vi "Teleop.vi"(10 "Match Info":T2={"Autonomous Elapsed Seconds"=0.0, "TeleOp Elapsed Seconds"=0.0, "Disabled Elapsed Seconds"=0.0, "Visited Autonomous"=FALSE, "Visited TeleOp"=FALSE, "Visited Disabled"=FALSE, "Autonomous Settings"={"Autonomous Style"=enum."Independent", "VI Refnum"=refnum}}, 11 "Call Context":T3) -> ()   [LabVIEW 2016]
doc: "This VI is called for each TeleOp packet received from the DS where the robot is not disabled. It is often used to read from the joysticks and update I/O or to update setpoints for timed control loops. It should complete and return within 20 milliseconds or it may miss DS packets."
uses:
  <vilib>/Rock Robotics/WPI/DriverStation/WPI_DriverStationDerivedRobotMode.ctl
  <vilib>/Rock Robotics/WPI/DriverStation/WPI_DriverStationMatch Info.ctl
  Robot Global Data.vi
  <vilib>/Rock Robotics/WPI/Utilities/WPI_GetSetVariantRefNum.vi
  <vilib>/Rock Robotics/WPI/Solenoid/Deprecated/WPI_SolenoidSetBool.vi
  <vilib>/Rock Robotics/Network Tables/NT Write Number.vi
  <vilib>/Rock Robotics/Network Tables/NT Write Boolean.vi
  <vilib>/addons/control/pid/pid.llb/PID (DBL).vi
  navX Library v2/navX Library v2.lvlib
  <vilib>/addons/control/pid/NI_PID_pid.lvlib
panel:
  in  "MOE":dbl=25.0 format="%#_13g"
  in  "Center":dbl=180.0 format="%#_13g"
  out "out left":dbl
  out "out right":dbl
  in  "Pid Factor":dbl=8400.0
  in  "Mode":bool=TRUE
  in  "output range":cluster{"output high":dbl, "output low":dbl}={"output high"=1.0, "output low"=-1.0} {"output low" format="%.2f"; "output high" format="%.2f"}
  in  "PID gains":T1={"proportional gain (Kc)"=0.00021, "integral time (Ti, min)"=15.0, "derivative time (Td, min)"=0.0} {"derivative time (Td, min)" format="%.6f"; "integral time (Ti, min)" format="%.6f"; "proportional gain (Kc)" format="%.6f"}
  out "Left":dbl(graph)
  out "Right":dbl(graph)
  out "Encoder Right":dbl(graph)
  out "Encoder Left":dbl(graph)
  in  "Speed":dbl=0.45 format="%#_13g"
  out "Out Left":dbl(graph)
  out "Out Right":dbl(graph)
  out "Shooter":cluster{"Sensor Velocity":dbl, dbl, dbl}(graph)
  in  "ShooterRPM":dbl
  in  "P":dbl=0.5 format="%#_13g"
  in  "I":dbl format="%#_13g"
  in  "D":dbl format="%#_13g"
  in  "F":dbl=0.005212 format="%#_13g"
  in  "I Zone":dbl format="%#_13g"
  in  "Ramp Rate":dbl format="%#_13g"
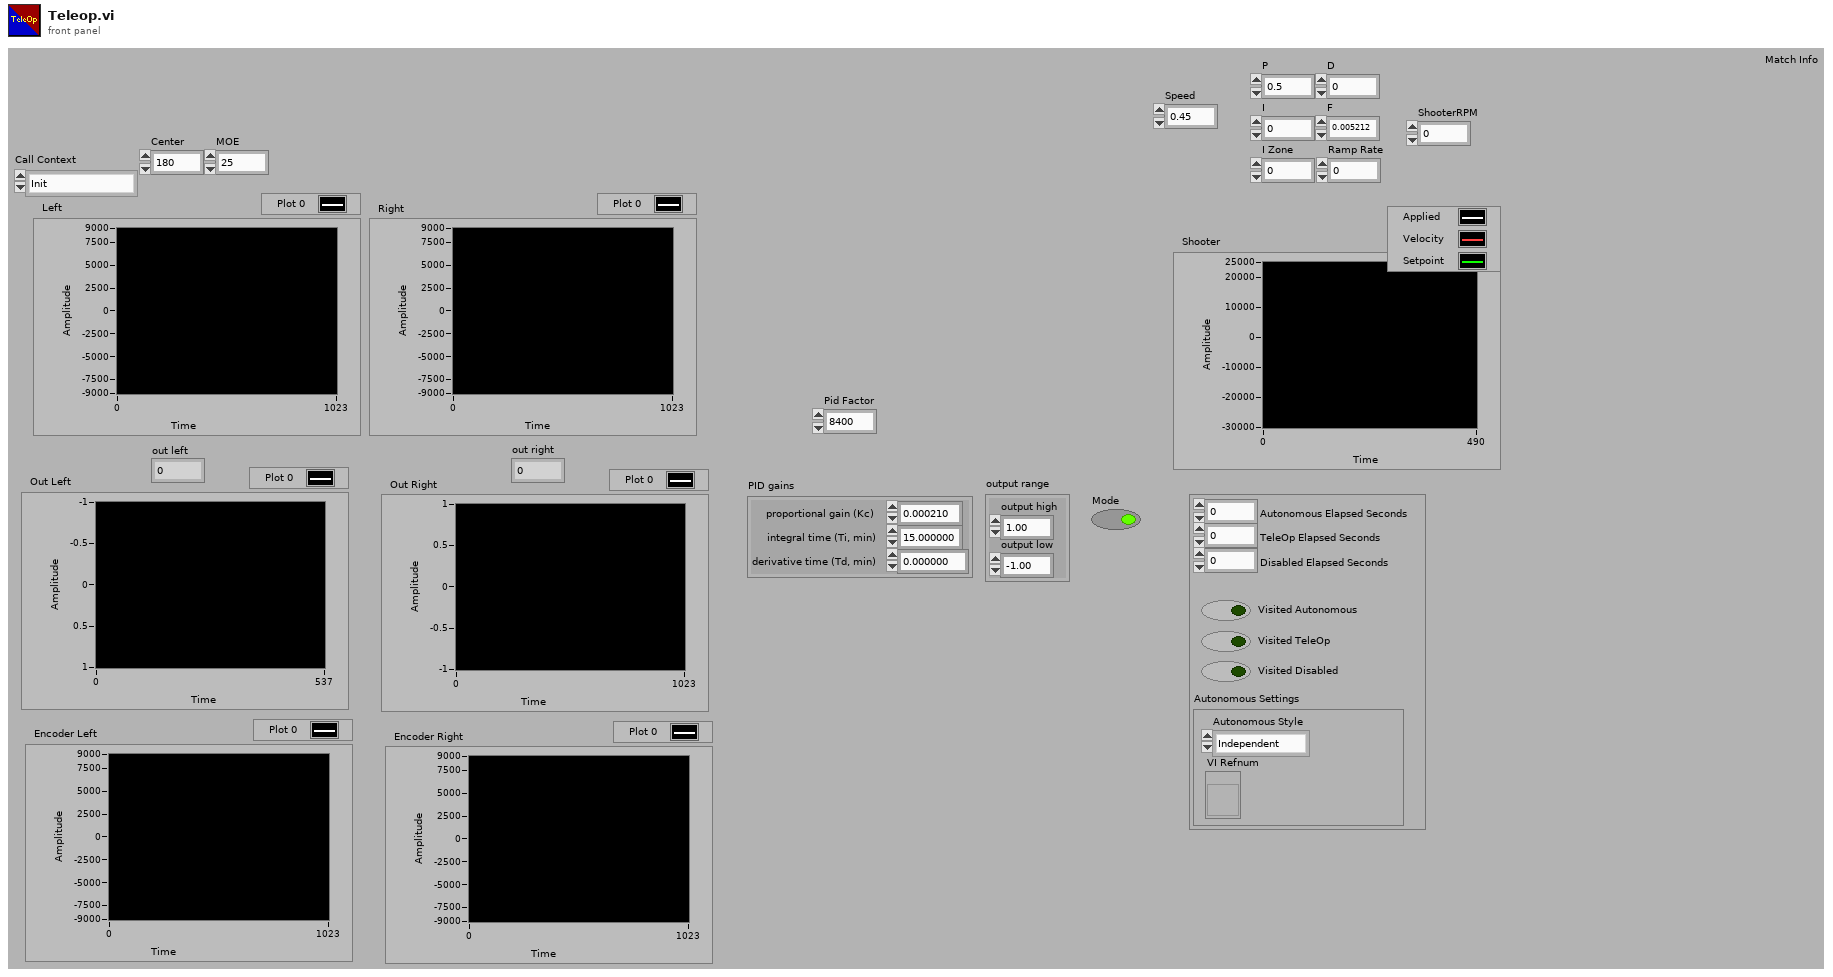
[diagram p1: front panel]
types:
  T1 = cluster{"proportional gain (Kc)":dbl, "integral time (Ti, min)":dbl, "derivative time (Td, min)":dbl}
  T2 = typedef "WPI_DriverStationMatch Info.ctl" = cluster{"Autonomous Elapsed Seconds":dbl, "TeleOp Elapsed Seconds":dbl, "Disabled Elapsed Seconds":dbl, "Visited Autonomous":bool, "Visited TeleOp":bool, "Visited Disabled":bool, "Autonomous Settings":cluster{"Autonomous Style":enum16{"Iterative", "Independent"}, "VI Refnum":refnum<vi>}}
  T3 = typedef "WPI_DriverStationDerivedRobotMode.ctl" = enum16{"Init", "Execute", "Stop"}
  T4 = typedef "WPI_SolenoidDevRef.ctl" = cluster{"DevStatus":errorcluster, "Pneumatics Control Module":u8, "Forward Solenoid Channel":T5, "Reverse Solenoid Channel":T5}
  T5 = typedef "WPI_SolenoidChannel.ctl" = enum8{"Solenoid 0", "Solenoid 1", "Solenoid 2", "Solenoid 3", "Solenoid 4", "Solenoid 5", "Solenoid 6", "Solenoid 7", "Invalid"}
  T6 = typedef "WPI_JoystickDevRef.ctl" = cluster{"Device":T7}
  T7 = typedef "WPI_JoystickDeviceEnum.ctl" = enum16{"USB 0", "USB 1", "USB 2", "USB 3", "USB 4", "USB 5"}
  T8 = cluster{"Buttons[0]":bool, "Buttons[1]":bool, "Buttons[2]":bool, "Buttons[3]":bool, "Buttons[4]":bool, "Buttons[5]":bool, "Buttons[6]":bool, "Buttons[7]":bool, "Buttons[8]":bool}
  T9 = cluster{"Axes[0]":dbl, "Axes[1]":dbl, "Axes[2]":dbl, "Axes[3]":dbl, "Axes[4]":dbl, "Axes[5]":dbl, "Axes[6]":dbl, "Axes[7]":dbl, "Axes[8]":dbl}
  T10 = typedef "navX Library v2.lvlib/Z900_navX_DeviceTypeDef.ctl" = cluster{"Interface":cluster{"Protocol":T11, "Update Rate (4Hz-100Hz)":u8, "navX Open TypeDef":variant}, "Notify Packet":refnum<notifier>, "Loop VI Refnum":refnum<vi>, "Ready to Close Occurrence Refnum":refnum<k4>}
  T11 = typedef "navX Library v2.lvlib/Z900_navX_ProtocolTypeDef.ctl" = enum16{"SERIAL", "I2C", "SPI"}
  T12 = cluster{"Velocity X":dbl, "Velocity Y":dbl, "Velocity Z":dbl, "Displacement X":dbl, "Displacement Y":dbl, "Displacement Z":dbl}
  T13 = cluster{"LinearAcceleration X":dbl, "LinearAcceleration Y":dbl, "LinearAcceleration Z":dbl}
  T14 = cluster{"Yaw":dbl, "Roll":dbl, "Pitch":dbl, "Heading":dbl, "Fused Heading":dbl}
  T15 = typedef "WPI_MotorControlDeviceRef.ctl" = cluster{"DeviceStatus":errorcluster, "Type":T16, "PWM":cluster{"PWM Channel":T17, "DeadBand":T18}, "CAN":cluster{"Device Number":u8, "SetOutput VI Ref":variant, "GetOutput VI Ref":variant, "Enable VI Ref":variant, "Disable VI Ref":variant, "Data":variant}, "Invert":bool}
  T16 = typedef "WPI_MotorControlType.ctl" = enum16{"PWM", "CAN"}
  T17 = typedef "FPGA_DIOPWMChannel.ctl" = enum8{"PWM 0", "PWM 1", "PWM 2", "PWM 3", "PWM 4", "PWM 5", "PWM 6", "PWM 7", "PWM 8", "PWM 9", "PWM MXP 0", "PWM MXP 1", "PWM MXP 2", "PWM MXP 3", "PWM MXP 4", "PWM MXP 5", "PWM MXP 6", "PWM MXP 7", "PWM MXP 8", "PWM MXP 9", "Invalid"}
  T18 = typedef "WPI_PWMDeadband.ctl" = cluster{"Name":string, "maxPositivePwm":i32, "minPositivePwm":i32, "centerPwm":i32, "maxNegativePwm":i32, "minNegativePwm":i32, "angularRange":u16}
  T19 = typedef "WPI_CANTalonSRX_GlobalStatus.ctl" = cluster{"Applied Throttle":dbl, "Module Enabled":bool, "CAN Error":errorcluster, "Closed Loop Error":dbl, "Forward Limit Switch Closed":bool, "Reverse Limit Switch Closed":bool, "Sensor Position":dbl, "Sensor Velocity":dbl, "Current":dbl, "Sticky Fault - Over Temp":bool, "Sticky Fault - Under Voltage":bool, "Sticky Fault - Forward Limit":bool, "Sticky Fault - Reverse Limit":bool, "Sticky Fault - Forward Soft Limit":bool, "Sticky Fault - Reverse Soft Limit":bool, "Brake is Enabled":bool, "Encoder Position":dbl, "Encoder Velocity":dbl, "Encoder Index Count":dbl, "Encoder A Pin State":bool, "Encoder B Pin State":bool, "Encoder Index Pin State":bool, "Analog In":dbl, "Analog In Velocity":dbl, "Temperature (C)":dbl, "Battery Voltage":dbl, "Control 5 Is Supported":bool, "Current Profile Slot Select":dbl, "Pos Div 8":bool, "Vel Div 4":bool, "Pulse Width Position":i32, "Pulse Width Velocity":i32, "Pulse Width Rise To Rise (us)":i32, "Pulse Width Rise To Fall (us)":i32, "Mot Prof Active Is Under Run":bool, "Mot Prof Active Has Under Run":bool, "Mot Prof Active Is Last":bool, "Mot Prof Active Velocity Only":bool, "Mot Prof Active Is Valid":bool, "Mot Prof Buffer Is Full":bool, "Mot Prof Active Profile Slot Select":i32, "Mot Prof NextID":i32, "Mot Prof Count":i32, "Mot Prof Active Velocity":dbl, "Mot Prof Active Position":dbl, "Mot Prof Output Enable":i32}
  T20 = cluster{dbl, "Sensor Velocity":dbl, "ShooterRPM":dbl}
  T21 = typedef "WPI_EncoderDevRef.ctl" = cluster{"DevStatus":errorcluster, "EncoderIndex":T22, "CounterIndex":T23, "DistancePerCount":dbl, "Decoding Type":T24}
  T22 = typedef "FPGA_EncoderIdx.ctl" = enum8{"Enc 0", "Enc 1", "Enc 2", "Enc 3", "Enc 4", "Enc 5", "Enc 6", "Enc 7", "Invalid"}
  T23 = typedef "FPGA_CounterCtrSystemIndex.ctl" = enum8{"Ctr 0", "Ctr 1", "Ctr 2", "Ctr 3", "Ctr 4", "Ctr 5", "Ctr 6", "Ctr 7", "Invalid"}
  T24 = typedef "WPI_EncoderType.ctl" = enum16{"1x", "2x", "4x"}
  T25 = typedef "WPI_RobotDriveDevRef.ctl" = cluster{"DevStatus":errorcluster, "Motors[]":T15[], "Square Inputs":bool, "Max Output":dbl}
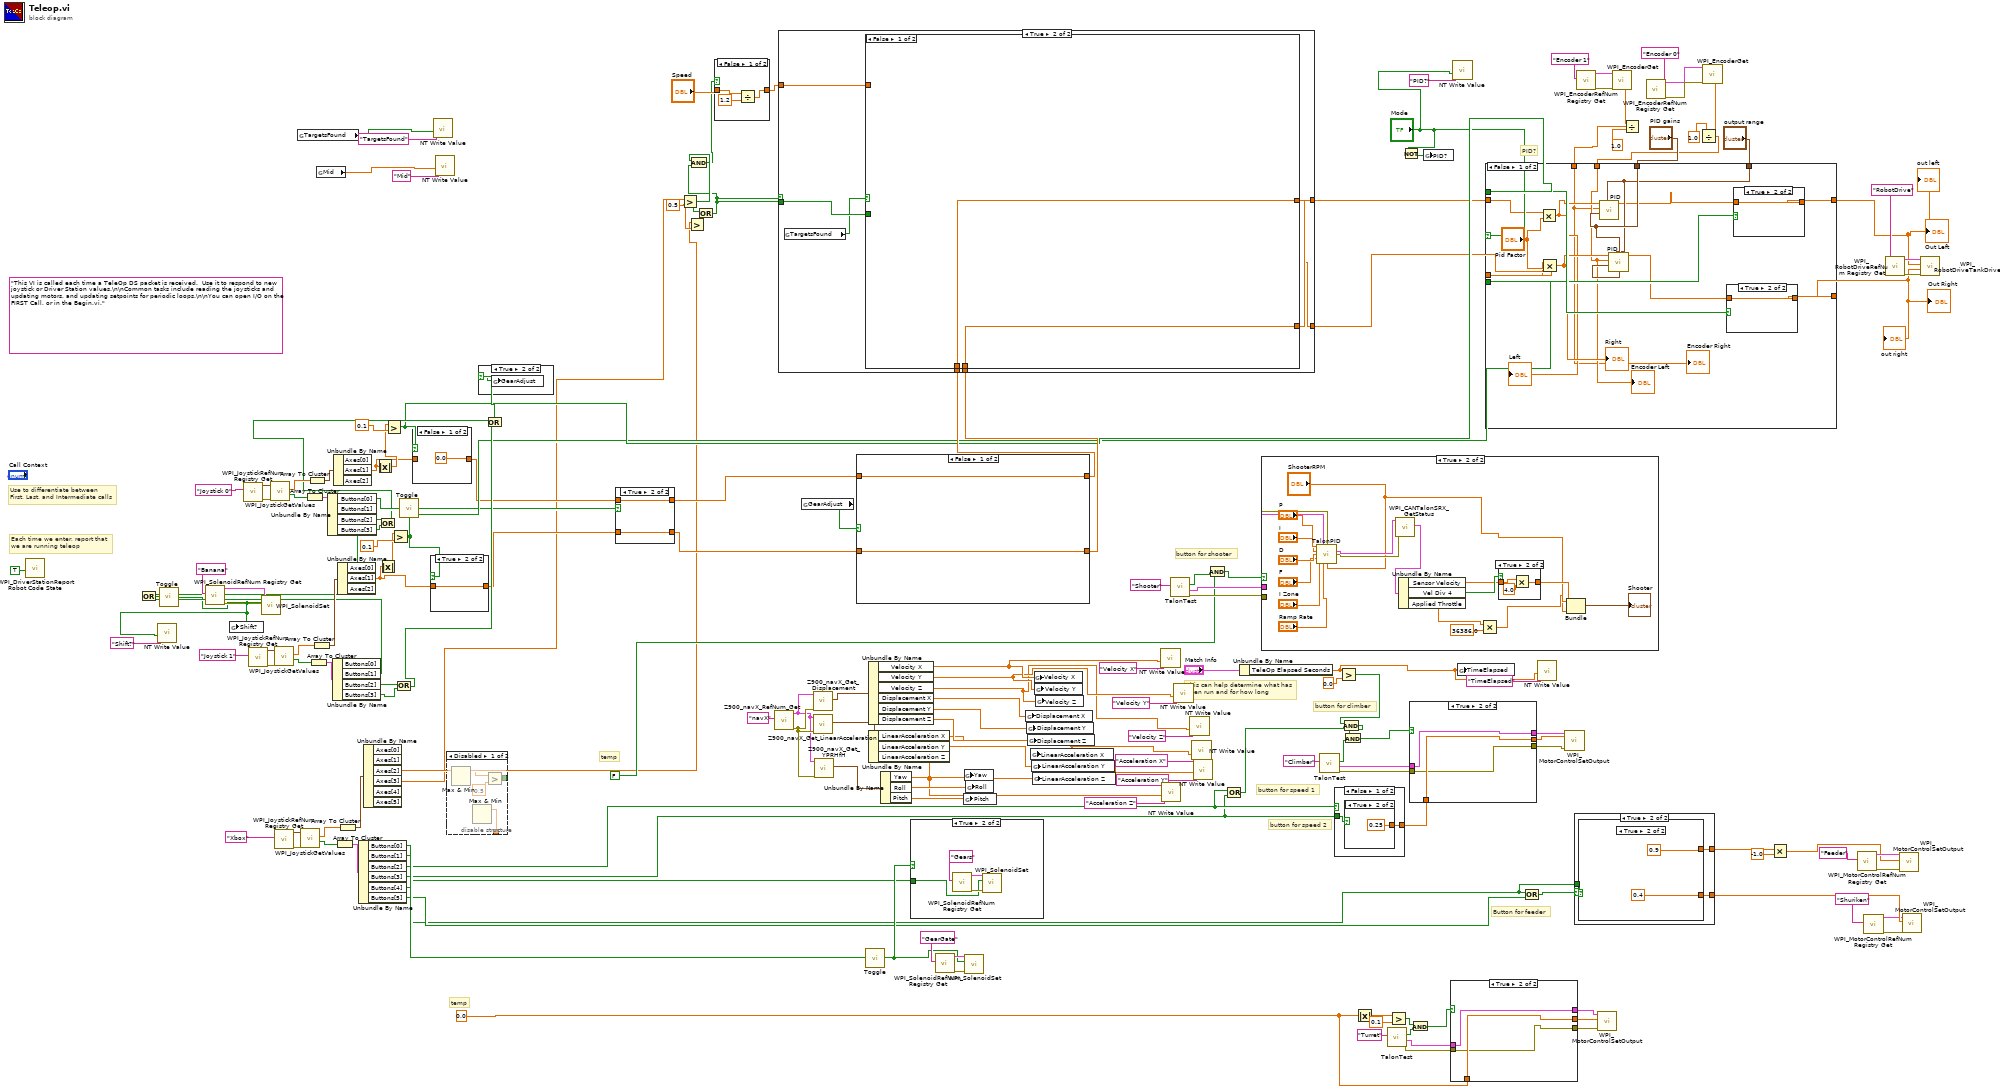
[diagram p0: block diagram]
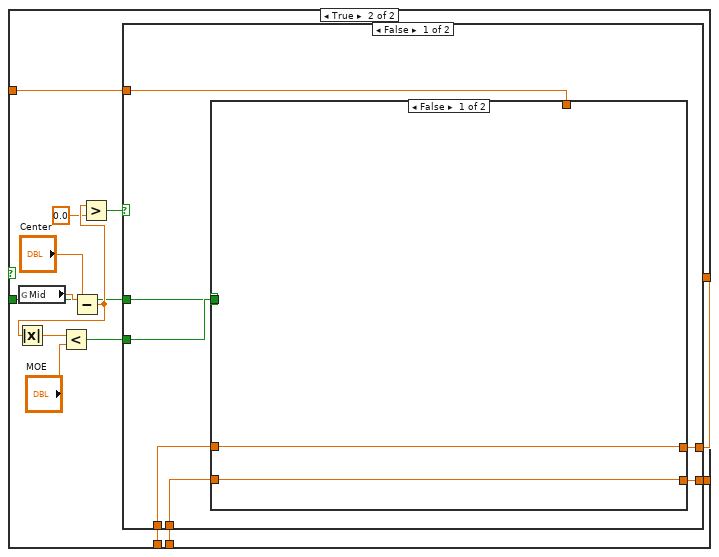
[diagram p4: hidden frame]
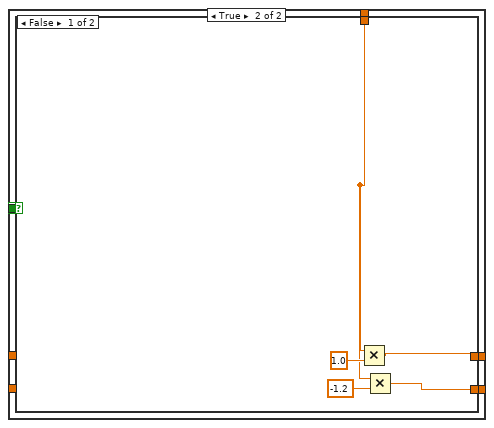
[diagram p5: hidden frame]
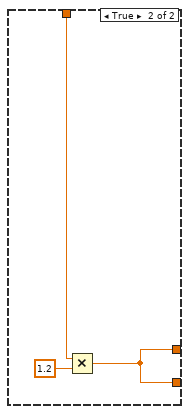
[diagram p6: hidden frame]
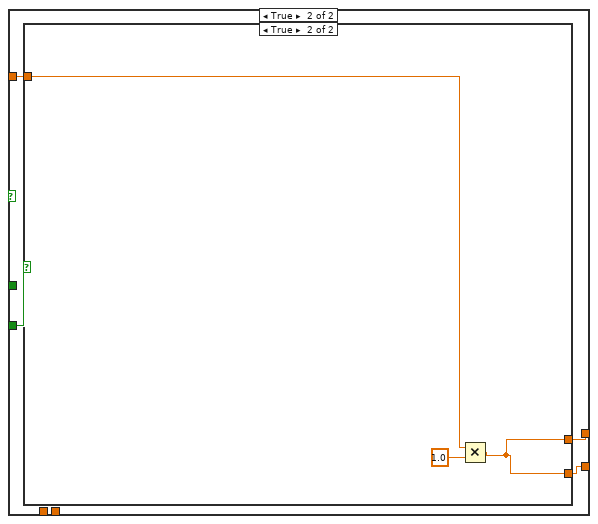
[diagram p7: hidden frame]
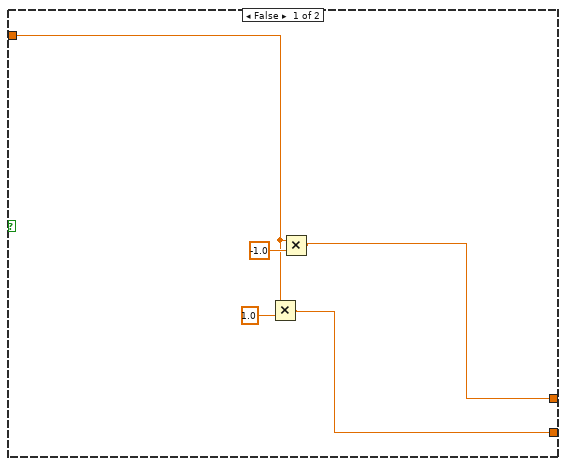
[diagram p8: hidden frame]
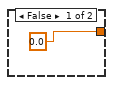
[diagram p9: hidden frame]
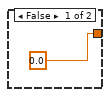
[diagram p10: hidden frame]
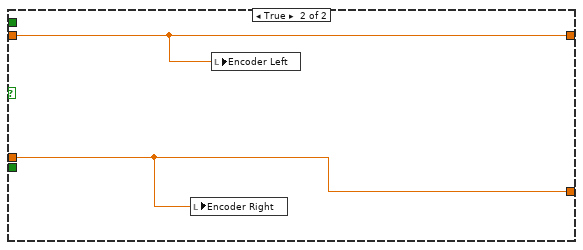
[diagram p11: hidden frame]
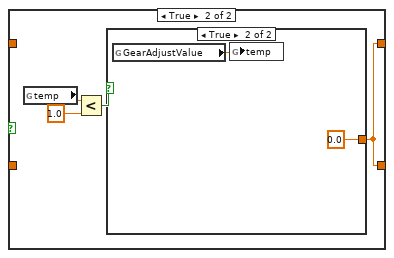
[diagram p14: hidden frame]
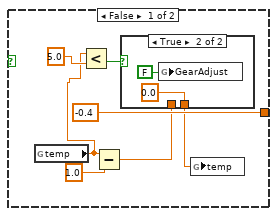
[diagram p15: hidden frame]
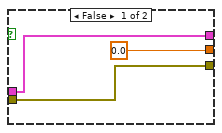
[diagram p17: hidden frame]
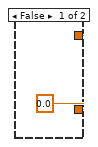
[diagram p19: hidden frame]
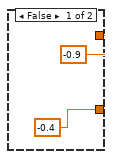
[diagram p20: hidden frame]
diagram:
  w32 = 0.5 ("y")
  w76 = 0.0
  (unwired) "This VI is called each time a TeleOp DS packet is received.  Use it to respond to new joystick or Driver Station values.\n\nCommon tasks include reading the joysticks and updating motors, and updating setpoints for periodic loops.\n\nYou can open I/O on the FIRST Call, or in the Begin.vi."
  # "PID?"
  # "temp"
  # "temp"
  # "Button for feeder"
  # "button for speed 2"
  # "button for speed 1"
  # "button for climber"
  # "button for shooter"
  # "Each time we enter, report that\nwe are running teleop"
  # "Use to differentiate between\nFirst, Last, and Intermediate calls"
  # "This can help determine what has\nbeen run and for how long"
  n1 = call <vilib>:"WPI_DriverStationReport Robot Code State.vi"("TeleOp"=TRUE ("Autonomous")) -> ()  [unwired: 10 in, 1 out]
  n2 = call <vilib>:"WPI_SolenoidRefNum Registry Get.vi"("refnum name"="Banana") -> ("error out"=w40:errorcluster, "SolenoidDevRef"=w39:T4)  [unwired: 9 in]
  n3 = call <vilib>:"WPI_JoystickRefNum Registry Get.vi"("refnum name"="Joystick 0") -> ("error out"=w169:errorcluster, "JoystickDevRef"=w168:T6)  [unwired: 9 in]
  n4 = call <vilib>:"WPI_JoystickRefNum Registry Get.vi"("refnum name"="Joystick 1") -> ("error out"=w161:errorcluster, "JoystickDevRef"=w160:T6)  [unwired: 9 in]
  n5 = call <vilib>:"WPI_JoystickGetValues.vi"("error in (no error)"=w169, "JoystickDevRef"=w168) -> ("Buttons"=w165:bool[], "Axes"=w166:dbl[])  [unwired: 5 in, 3 out]
  n6 = call <vilib>:"WPI_JoystickRefNum Registry Get.vi"("refnum name"="Xbox") -> ("error out"=w123:errorcluster, "JoystickDevRef"=w122:T6)  [unwired: 9 in]
  n7 = call <vilib>:"WPI_JoystickGetValues.vi"("error in (no error)"=w161, "JoystickDevRef"=w160) -> ("Buttons"=w157:bool[], "Axes"=w158:dbl[])  [unwired: 5 in, 3 out]
  n8 = global read "Robot Global Data.vi" "TargetsFound"() -> (w3:bool)
  n9 = call <vilib>:"WPI_JoystickGetValues.vi"("error in (no error)"=w123, "JoystickDevRef"=w122) -> ("Buttons"=w119:bool[], "Axes"=w120:dbl[])  [unwired: 5 in, 3 out]
  n10 = Array To Cluster(array=w165) -> (cluster=w163:T8)
  n11 = Array To Cluster(array=w166) -> (cluster=w164:T9)
  n12 = Array To Cluster(array=w157) -> (cluster=w155:T8)
  n13 = Array To Cluster(array=w158) -> (cluster=w156:T9)
  n14 = global read "Robot Global Data.vi" "Mid"() -> (w1:dbl)
  n15 = Unbundle By Name(w163) -> ("Buttons[0]"=w149:bool, "Buttons[1]"=w35:bool, "Buttons[2]"=w82:bool, "Buttons[3]"=w81:bool)
  n16 = Unbundle By Name(w155) -> ("Buttons[1]"=w36:bool, "Buttons[2]"=w84:bool, "Buttons[3]"=w83:bool)  [unwired: 1 out]
  n17 = Or(x=w35, y=w36) -> (x .or. y?=w37:bool)
  n18 = call "Toggle.vi"("Input"=w37) -> ("Output"=w17:bool)
  n19 = call-poly <vilib>:"NT Write Value.vi"("Boolean"=w17, "Name"="Shift?") -> ()  [unwired: 9 in, 1 out]
  n20 = global write "Robot Global Data.vi" "Shift?"(w17) -> ()
  n21 = call-poly <vilib>:"WPI_SolenoidSet.vi"("error in (no error)"=w40, "Value"=w17, "SolenoidDevRef"=w39) -> ()  [unwired: 7 in, 2 out]
  n22 = Unbundle By Name(w164) -> ("Axes[1]"=w150:dbl)  [unwired: 2 out]
  n23 = Array To Cluster(array=w119) -> (cluster=w117:T8)
  n24 = Unbundle By Name(w156) -> ("Axes[1]"=w152:dbl)  [unwired: 2 out]
  n25 = Array To Cluster(array=w120) -> (cluster=w118:T9)
  n26 = Unbundle By Name(w117) -> ("Buttons[0]"=w116:bool, "Buttons[1]"=w115:bool, "Buttons[2]"=w114:bool, "Buttons[3]"=w113:bool, "Buttons[4]"=w110:bool, "Buttons[5]"=w111:bool)
  n27 = Unbundle By Name(w118) -> ("Axes[2]"=w25:dbl, "Axes[3]"=w24:dbl)  [unwired: 4 out]
  n28 = Absolute Value(x=w150) -> (abs(x)=w151:dbl)
  n29 = Or(x=w82, y=w81) -> (x .or. y?=w80:bool)
  n30 = Absolute Value(x=w152) -> (abs(x)=w153:dbl)
  n31 = Greater?(x=w151, y=0.1 ("x")) -> (0:w66:bool)
  n32 = Greater?(x=w153, y=0.1 ("x")) -> (0:w65:bool)
  n33 = Or(x=w84, y=w83) -> (x .or. y?=w79:bool)
  n34 = call "Toggle.vi"("Input"=w149) -> ("Output"=w60:bool)
  n35 = case shown="False" w66 {
    tunnel: w150 -> [_ w172]
    tunnel: [0.0 w172] -> w63
    frame False {
    }
    frame True {
    }
  }
  n36 = case shown="True" w65 {
    tunnel: w152 -> [_ w174]
    tunnel: [0.0 w174] -> w64
    frame False {
    }
    frame True {
    }
  }
  n37 = call-poly <vilib>:"NT Write Value.vi"("Boolean"=w3, "Name"="TargetsFound") -> ()  [unwired: 9 in, 1 out]
  n38 = call-poly <vilib>:"NT Write Value.vi"("Numeric"=w1, "Name"="Mid") -> ()  [unwired: 9 in, 1 out]
  n39 = disable-structure shown="Disabled" {
    disable-tunnel: [w176 _] -> _
    disable-tunnel: [w175 _] -> _
    frame Disabled {
      n40 = Max & Min() -> (max(x,y)=w178:dbl)  [unwired: 2 in, 1 out]
      n41 = Max & Min() -> (max(x,y)=w175:dbl)  [unwired: 2 in, 1 out]
      n42 = Greater?(x=w178, y=0.5) -> (0:w176:bool)
    }
    frame Enabled {
    }
  }
  n43 = Or(x=w80, y=w79) -> (x .or. y?=w77:bool)
  n44 = case shown="True" w77 {
    selector: w77 -> [_ w179]
    frame False {
    }
    frame True {
      n45 = global write "Robot Global Data.vi" "GearAdjust"(w179) -> ()
    }
  }
  n46 = case shown="True" w60 {
    tunnel: w63 -> [w181 w186]
    tunnel: w64 -> [w180 w185]
    tunnel: [w184 w186] -> w62
    tunnel: [w183 w185] -> w61
    frame False {
      w182 = -1.0
      n47 = Multiply(x=w182, y=w181) -> (x*y=w183:dbl)
      n48 = Multiply(x=w180, y=w182) -> (x*y=w184:dbl)
    }
    frame True {
    }
  }
  n49 = Greater?(x=w24, y=w32) -> (0:w30:bool)
  n50 = Greater?(x=w25, y=w32) -> (0:w31:bool)
  n51 = Or(x=w30, y=w31) -> (x .or. y?=w29:bool)
  n52 = And(x=w30, y=w29) -> (x .and. y?=w26:bool)
  n53 = case shown="False" w26 {
    tunnel: [w189 w190] -> w27
    tunnel: "Speed" -> [w188 w190]
    frame False {
      n54 = Divide(x=w188, y=1.2) -> (x/y=w189:dbl)
    }
    frame True {
    }
  }
  n55 = call "Z900_navX_RefNum_Get.vi"("refnum name"="navX") -> ("error out"=w147:errorcluster, "navX Device"=w146:T10)  [unwired: 9 in]
  n56 = global read "Robot Global Data.vi" "GearAdjust"() -> (w78:bool)
  n57 = call "Z900_navX_Get_Displacement.vi"("error in (no error)"=w147, "navX Device"=w146) -> ("Displacement"=w143:T12)  [unwired: 6 in, 3 out]
  n58 = call "Z900_navX_Get_LinearAcceleration.vi"("error in (no error)"=w147, "navX Device"=w146) -> ("Linear Acceleration"=w144:T13)  [unwired: 6 in, 3 out]
  n59 = call "Z900_navX_Get_YPRHfH.vi"("error in (no error)"=w147, "navX Device"=w146) -> ("YRPHfH"=w145:T14)  [unwired: 6 in, 3 out]
  n60 = case shown="False" w78 {
    tunnel: w62 -> [w192 _]
    tunnel: w61 -> [w191 _]
    tunnel: [w192 w193] -> w71
    tunnel: [w191 w193] -> w70
    frame False {
    }
    frame True {
      n61 = global read "Robot Global Data.vi" "temp"() -> (w196:dbl)
      n62 = Less?(x=w196, y=1.0) -> (x < y?=w194:bool)
      n63 = case shown="True" w194 {
        tunnel: [-0.4 0.0] -> w193
        frame False {
          n64 = global read "Robot Global Data.vi" "temp"() -> (w199:dbl)
          n65 = Less?(x=w199, y=5.0 ("x")) -> (x < y?=w200:bool)
          n66 = Subtract(x=w199, y=1.0) -> (x-y=w197:dbl)
          n67 = case shown="True" w200 {
            tunnel: [w204 0.0] -> w198
            tunnel: w197 -> [w204 _]
            frame False {
            }
            frame True {
              n68 = global write "Robot Global Data.vi" "GearAdjust"(FALSE) -> ()
            }
          }
          n69 = global write "Robot Global Data.vi" "temp"(w198) -> ()
        }
        frame True {
          n70 = global read "Robot Global Data.vi" "GearAdjustValue"() -> (w208:dbl)
          n71 = global write "Robot Global Data.vi" "temp"(w208) -> ()
        }
      }
    }
  }
  n72 = case shown="True" w29 {
    tunnel: w71 -> [w210 w217]
    tunnel: w70 -> [w209 w216]
    tunnel: w29 -> [_ w215]
    tunnel: [w210 w213] -> w33
    tunnel: [w209 w212] -> w34
    tunnel: w27 -> [_ w211]
    frame False {
    }
    frame True {
      n73 = global read "Robot Global Data.vi" "TargetsFound"() -> (w214:bool)
      n74 = case shown="False" w214 {
        tunnel: w217 -> [w219 w228]
        tunnel: w216 -> [w218 w227]
        tunnel: [w218 w226] -> w213
        tunnel: [w219 w225] -> w212
        tunnel: w215 -> [_ w221]
        tunnel: w211 -> [_ w220]
        frame False {
        }
        frame True {
          n75 = global read "Robot Global Data.vi" "Mid"() -> (w233:dbl)
          n76 = Subtract(x=w233, y="Center") -> (x-y=w223:dbl)
          n77 = Absolute Value(x=w223) -> (abs(x)=w231:dbl)
          n78 = Less?(x=w231, y="MOE") -> (x < y?=w229:bool)
          n79 = Greater?(x=w223, y=0.0) -> (0:w224:bool)
          n80 = case shown="False" w224 {
            tunnel: w229 -> [w240 w258]
            tunnel: w228 -> [w239 _]
            tunnel: w227 -> [w238 _]
            tunnel: [w237 w256] -> w226
            tunnel: [w236 w257] -> w225
            tunnel: w221 -> [w235 _]
            tunnel: w220 -> [w234 w255]
            frame False {
              n81 = case shown="False" w235 {
                tunnel: w240 -> [_ w246]
                tunnel: w239 -> [w242 _]
                tunnel: w238 -> [w241 _]
                tunnel: [w242 w245] -> w236
                tunnel: [w241 w244] -> w237
                tunnel: w234 -> [_ w243]
                frame False {
                }
                frame True {
                  n82 = case shown="False" w246 {
                    tunnel: [w251 w254] -> w245
                    tunnel: [w249 w254] -> w244
                    tunnel: w243 -> [w247 w252]
                    frame False {
                      n83 = Multiply(x=w247, y=1.0) -> (x*y=w251:dbl)
                      n84 = Multiply(x=w247, y=-1.2) -> (x*y=w249:dbl)
                    }
                    frame True {
                      n85 = Multiply(x=w252, y=1.2) -> (x*y=w254:dbl)
                    }
                  }
                }
              }
            }
            frame True {
              n86 = case shown="True" w258 {
                tunnel: [w263 w266] -> w257
                tunnel: [w261 w266] -> w256
                tunnel: w255 -> [w259 w264]
                frame False {
                  n87 = Multiply(x=w259, y=1.0) -> (x*y=w261:dbl)
                  n88 = Multiply(x=w259, y=-1.0) -> (x*y=w263:dbl)
                }
                frame True {
                  n89 = Multiply(x=w264, y=1.0) -> (x*y=w266:dbl)
                }
              }
            }
          }
        }
      }
    }
  }
  n90 = call "Toggle.vi"("Input"=w116) -> ("Output"=w124:bool)
  n91 = Unbundle By Name(w143) -> ("Velocity X"=w10:dbl, "Velocity Y"=w9:dbl, "Velocity Z"=w8:dbl, "Displacement X"=w59:dbl, "Displacement Y"=w58:dbl, "Displacement Z"=w57:dbl)
  n92 = Unbundle By Name(w144) -> ("LinearAcceleration X"=w7:dbl, "LinearAcceleration Y"=w6:dbl, "LinearAcceleration Z"=w5:dbl)
  n93 = Unbundle By Name(w145) -> ("Yaw"=w56:dbl, "Roll"=w55:dbl, "Pitch"=w54:dbl)
  n94 = case shown="True" w124 {
    tunnel: w115 -> [_ w267]
    frame False {
    }
    frame True {
      n95 = call <vilib>:"WPI_SolenoidRefNum Registry Get.vi"("refnum name"="Gears") -> ("error out"=w270:errorcluster, "SolenoidDevRef"=w269:T4)  [unwired: 9 in]
      n96 = call-poly <vilib>:"WPI_SolenoidSet.vi"("error in (no error)"=w270, "Value"=w267, "SolenoidDevRef"=w269) -> ()  [unwired: 7 in, 2 out]
    }
  }
  n97 = call <vilib>:"WPI_SolenoidRefNum Registry Get.vi"("refnum name"="GearGate") -> ("error out"=w127:errorcluster, "SolenoidDevRef"=w126:T4)  [unwired: 9 in]
  n98 = global write "Robot Global Data.vi" "Pitch"(w54) -> ()
  n99 = global write "Robot Global Data.vi" "Yaw"(w56) -> ()
  n100 = call-poly <vilib>:"WPI_SolenoidSet.vi"("error in (no error)"=w127, "Value"=w124, "SolenoidDevRef"=w126) -> ()  [unwired: 7 in, 2 out]
  n101 = global write "Robot Global Data.vi" "Roll"(w55) -> ()
  n102 = global write "Robot Global Data.vi" "Displacement X"(w59) -> ()
  n103 = global write "Robot Global Data.vi" "Displacement Y"(w58) -> ()
  n104 = global write "Robot Global Data.vi" "Displacement Z"(w57) -> ()
  n105 = global write "Robot Global Data.vi" "LinearAcceleration X"(w7) -> ()
  n106 = global write "Robot Global Data.vi" "LinearAcceleration Y"(w6) -> ()
  n107 = global write "Robot Global Data.vi" "LinearAcceleration Z"(w5) -> ()
  n108 = global write "Robot Global Data.vi" "Velocity X"(w10) -> ()
  n109 = global write "Robot Global Data.vi" "Velocity Y"(w9) -> ()
  n110 = global write "Robot Global Data.vi" "Velocity Z"(w8) -> ()
  n111 = call-poly <vilib>:"NT Write Value.vi"("Numeric"=w10, "Name"="Velocity X") -> ()  [unwired: 9 in, 1 out]
  n112 = call-poly <vilib>:"NT Write Value.vi"("Numeric"=w5, "Name"="Acceleration Z") -> ()  [unwired: 9 in, 1 out]
  n113 = call "TalonTest.vi"("Name"="Shooter") -> ("Output"=w137:bool, "Ref"=w141:T15, "error out"=w140:errorcluster)  [unwired: 7 in]
  n114 = call-poly <vilib>:"NT Write Value.vi"("Numeric"=w9, "Name"="Velocity Y") -> ()  [unwired: 9 in, 1 out]
  n115 = call-poly <vilib>:"NT Write Value.vi"("Numeric"=w8, "Name"="Velocity Z") -> ()  [unwired: 9 in, 1 out]
  n116 = call-poly <vilib>:"NT Write Value.vi"("Numeric"=w7, "Name"="Acceleration X") -> ()  [unwired: 9 in, 1 out]
  n117 = call-poly <vilib>:"NT Write Value.vi"("Numeric"=w6, "Name"="Acceleration Y") -> ()  [unwired: 9 in, 1 out]
  n118 = And(x=FALSE, y=w137) -> (x .and. y?=w138:bool)
  n119 = Or(x=w114, y=w113) -> (x .or. y?=w112:bool)
  n120 = Unbundle By Name("Match Info") -> ("TeleOp Elapsed Seconds"=w22:dbl)
  n121 = case shown="True" w138 {
    tunnel: w141 -> [_ w275]
    tunnel: w140 -> [_ w271]
    frame False {
    }
    frame True {
      n122 = call "TalonPID.vi"("P"="P", "Ref In"=w275, "Error in"=w271, "I"="I", "D"="D", "F"="F", "I Zone"="I Zone", "Ramp Rate"="Ramp Rate", "Output"="ShooterRPM") -> ("Ref Out"=w274:T15, "error out"=w273:errorcluster)  [unwired: 5 in]
      n123 = call <vilib>:"WPI_CANTalonSRX_GetStatus.vi"("error in (no error)"=w273, "CAN Talon SRX Ref"=w274) -> ("Talon SRX Status"=w289:T19)  [unwired: 7 in, 2 out]
      n124 = Unbundle By Name(w289) -> ("Sensor Velocity"=w287:dbl, "Vel Div 4"=w288:bool, "Applied Throttle"=w284:dbl)
      n125 = Multiply(x=w284, y=36386.0) -> (x*y=w283:dbl)
      n126 = case shown="True" w288 {
        tunnel: w287 -> [w290 w292]
        tunnel: [w290 w293] -> w282
        frame False {
        }
        frame True {
          n127 = Multiply(x=w292, y=4.0) -> (x*y=w293:dbl)
        }
      }
      n128 = Bundle(w283, "Sensor Velocity"=w282, "ShooterRPM"="ShooterRPM") -> (→"Shooter":T20)  [unwired: 1 in]
    }
  }
  n129 = call "TalonTest.vi"("Name"="Climber") -> ("Output"=w135:bool, "Ref"=w130:T15, "error out"=w129:errorcluster)  [unwired: 7 in]
  n130 = case shown="False" w114 {
    tunnel: [w295 w299] -> w128
    tunnel: w113 -> [w294 w298]
    frame False {
      n131 = case shown="True" w294 {
        tunnel: [0.0 0.25] -> w295
        frame False {
        }
        frame True {
        }
      }
    }
    frame True {
      n132 = case shown="True" w298 {
        tunnel: [0.75 1.0] -> w299
        frame False {
        }
        frame True {
        }
      }
    }
  }
  n133 = Greater?(x=w22, y=0.0) -> (0:w132:bool)
  n134 = And(x=w132, y=w112) -> (x .and. y?=w136:bool)
  n135 = And(x=w136, y=w135) -> (x .and. y?=w131:bool)
  n136 = Absolute Value(x=w76) -> (abs(x)=w103:dbl)
  n137 = call "TalonTest.vi"("Name"="Turret") -> ("Output"=w107:bool, "Ref"=w105:T15, "error out"=w104:errorcluster)  [unwired: 7 in]
  n138 = Greater?(x=w103, y=0.1) -> (0:w101:bool)
  n139 = Not(x="Mode") -> (.not. x?=w23:bool)
  n140 = case shown="True" w131 {
    tunnel: w130 -> [w303 w307]
    tunnel: w129 -> [w302 w305]
    tunnel: w128 -> [_ w306]
    tunnel: [w303 w307] -> w96
    tunnel: [0.0 w306] -> w97
    tunnel: [w302 w305] -> w95
    frame False {
    }
    frame True {
    }
  }
  n141 = And(x=w101, y=w107) -> (x .and. y?=w106:bool)
  n142 = global write "Robot Global Data.vi" "PID?"(w23) -> ()
  n143 = case shown="True" w106 {
    tunnel: w105 -> [w309 w313]
    tunnel: w104 -> [w308 w311]
    tunnel: w76 -> [_ w312]
    tunnel: [w309 w313] -> w100
    tunnel: [0.0 w312] -> w99
    tunnel: [w308 w311] -> w98
    frame False {
    }
    frame True {
    }
  }
  n144 = call-poly <vilib>:"NT Write Value.vi"("Boolean"="Mode", "Name"="PID?") -> ()  [unwired: 9 in, 1 out]
  n145 = global write "Robot Global Data.vi" "TimeElapsed"(w22) -> ()
  n146 = Or(x=w110, y=w111) -> (x .or. y?=w109:bool)
  n147 = call-poly <vilib>:"NT Write Value.vi"("Numeric"=w22, "Name"="TimeElapsed") -> ()  [unwired: 9 in, 1 out]
  n148 = call <vilib>:"WPI_MotorControlSetOutput.vi"("error in (no error)"=w95, "Output"=w97, "MotorControlDevRef"=w96) -> ()  [unwired: 6 in, 3 out]
  n149 = case shown="True" w109 {
    tunnel: w110 -> [_ w317]
    tunnel: [w314 w316] -> w87
    tunnel: [w314 w315] -> w94
    frame False {
      w314 = 0.0
    }
    frame True {
      n150 = case shown="True" w317 {
        tunnel: [-0.9 ("Output") 0.9 ("Output")] -> w316
        tunnel: [-0.4 ("Output") 0.4 ("Output")] -> w315
        frame False {
        }
        frame True {
        }
      }
    }
  }
  n151 = call <vilib>:"WPI_EncoderRefNum Registry Get.vi"("refnum name"="Encoder 1") -> ("error out"=w53:errorcluster, "EncoderDevRef"=w52:T21)  [unwired: 9 in]
  n152 = call <vilib>:"WPI_MotorControlSetOutput.vi"("error in (no error)"=w98, "Output"=w99, "MotorControlDevRef"=w100) -> ()  [unwired: 6 in, 3 out]
  n153 = call <vilib>:"WPI_EncoderGet.vi"("error in (no error)"=w53, "EncoderDevRef"=w52) -> ("Rate"=w43:dbl)  [unwired: 4 in, 5 out]
  n154 = Divide(x=w43, y=1.0) -> (x/y=w46:dbl)
  n155 = call <vilib>:"WPI_EncoderRefNum Registry Get.vi"("refnum name"="Encoder 0") -> ("error out"=w50:errorcluster, "EncoderDevRef"=w49:T21)  [unwired: 9 in]
  n156 = call <vilib>:"WPI_EncoderGet.vi"("error in (no error)"=w50, "EncoderDevRef"=w49) -> ("Rate"=w45:dbl)  [unwired: 4 in, 5 out]
  n157 = Divide(x=w45, y=1.0) -> (x/y=w47:dbl)
  n158 = case shown="False" "Mode" {
    tunnel: w33 -> [w327 w342]
    tunnel: w34 -> [w326 w341]
    tunnel: w46 -> [w322 _]
    tunnel: w47 -> [w323 _]
    tunnel: "PID gains" -> [w336 _]
    tunnel: "output range" -> [w335 _]
    tunnel: w66 -> [w332 _]
    tunnel: w65 -> [w331 _]
    tunnel: [w333 w341] -> w68
    tunnel: [w334 w342] -> w41
    frame False {
      n159 = Multiply(x=w327, y="Pid Factor") -> (x*y=w324:dbl)
      "Left" <- w324
      n160 = Multiply(x=w326, y="Pid Factor") -> (x*y=w325:dbl)
      "Right" <- w325
      n161 = call-poly <vilib>:"PID.vi"("output range"=w335, "PID gains"=w336, "process variable"=w322, "setpoint"=w324) -> ("output"=w330:dbl)  [unwired: 6 in, 1 out]
      n162 = call-poly <vilib>:"PID.vi"("output range"=w335, "PID gains"=w336, "process variable"=w323, "setpoint"=w325) -> ("output"=w329:dbl)  [unwired: 6 in, 1 out]
      n163 = case shown="True" w332 {
        tunnel: w329 -> [_ w338]
        tunnel: [0.0 w338] -> w333
        frame False {
        }
        frame True {
        }
      }
      n164 = case shown="True" w331 {
        tunnel: w330 -> [_ w340]
        tunnel: [0.0 w340] -> w334
        frame False {
        }
        frame True {
        }
      }
      "Encoder Right" <- w322
      "Encoder Left" <- w323
    }
    frame True {
      n165 = local write "Encoder Right"(w341) -> ()
      n166 = local write "Encoder Left"(w342) -> ()
    }
  }
  "Out Right" <- w68
  "Out Left" <- w41
  "out right" <- w68
  "out left" <- w41
  n167 = Multiply(x=w87, y=-1.0) -> (x*y=w85:dbl)
  n168 = call <vilib>:"WPI_MotorControlRefNum Registry Get.vi"("refnum name"="Feeder") -> ("error out"=w88:errorcluster, "MotorControlDevRef"=w89:T15)  [unwired: 9 in]
  n169 = call <vilib>:"WPI_MotorControlRefNum Registry Get.vi"("refnum name"="Shuriken") -> ("error out"=w90:errorcluster, "MotorControlDevRef"=w91:T15)  [unwired: 9 in]
  n170 = call <vilib>:"WPI_RobotDriveRefNum Registry Get.vi"("refnum name"="RobotDrive") -> ("error out"=w74:errorcluster, "RobotDriveDevRef"=w73:T25)  [unwired: 9 in]
  n171 = call <vilib>:"WPI_MotorControlSetOutput.vi"("error in (no error)"=w88, "Output"=w85, "MotorControlDevRef"=w89) -> ()  [unwired: 6 in, 3 out]
  n172 = call <vilib>:"WPI_MotorControlSetOutput.vi"("error in (no error)"=w90, "Output"=w94, "MotorControlDevRef"=w91) -> ()  [unwired: 6 in, 3 out]
  n173 = call <vilib>:"WPI_RobotDriveTankDrive.vi"("error in (no error)"=w74, "Right axis value"=w68, "Left axis value"=w41, "RobotDriveDevRef"=w73) -> ()  [unwired: 5 in, 3 out]
